vi "getAll.vi"(8 "error in (no error)":errorcluster, 11 "Example Instrument in":refnum<class "ExampleInstrument.lvclass">) -> (0 "error out":errorcluster, 2 "getAll":variant, 3 "Example Instrument out":refnum<class "ExampleInstrument.lvclass">)   [LabVIEW 2016, in "ExampleInstrument.lvclass"]
uses:
  ExampleInstrument.lvclass
  Typedefs/ExampleInstrument.getAll--Cluster.ctl
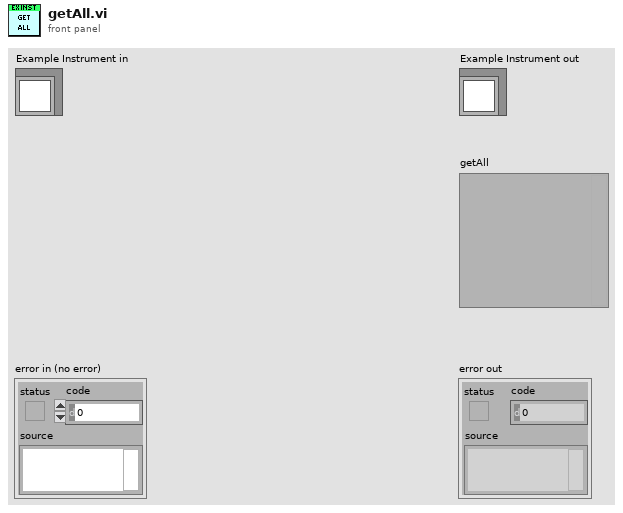
[diagram p1: front panel]
types:
  T1 = typedef "ExampleInstrument.lvclass/ExampleInstrument.getAll--Cluster.ctl" = cluster{"Levy 1":dbl, "Logger SMO":dbl, "SMO Boolean":bool, "SMO String":string}
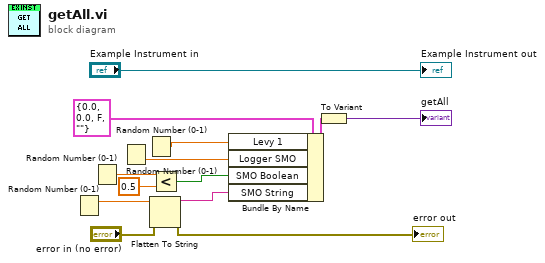
[diagram p0: block diagram]
diagram:
  n1 = Random Number (0-1)() -> (number: 0 to 1=w5:dbl)
  n2 = Random Number (0-1)() -> (number: 0 to 1=w8:dbl)
  n3 = Random Number (0-1)() -> (number: 0 to 1=w9:dbl)
  n4 = Random Number (0-1)() -> (number: 0 to 1=w10:dbl)
  n5 = Flatten To String(anything=w5, error in (no error)="error in (no error)") -> (data string=w4:string, error out=→"error out":errorcluster)  [unwired: 2 in, 1 out]
  n6 = Less?(x=w8, y=0.5) -> (x < y?=w7:bool)
  n7 = Bundle By Name(cluster=T1 {"Levy 1"=0.0, "Logger SMO"=0.0, "SMO Boolean"=FALSE, "SMO String"=""} ("getAll"), "Levy 1"=w10, "Logger SMO"=w9, "SMO Boolean"=w7, "SMO String"=w4) -> (w11:T1)
  n8 = To Variant(anything=w11) -> (Variant=→"getAll":variant)
  "Example Instrument out" <- "Example Instrument in"
